vi "dialog.two_button_lua.vi"(5 "LuaVIEW reference":T1) -> (15 "error out":errorcluster)   [LabVIEW 2012]
doc: "Display a two-button dialog with a message. Returns when either button is selected, the dialog window is closed, or the Escape key is pressed. When the left button is selected, the result Boolean returns true. Otherwise false is returned.\n\nThe shown dialog is functionally identical to the standard LabVIEW \"Two Button Dialog\". The standard dialog is not used because, at least up to LabVIEW version 7.1, it has the nasty property that it blocks the user interface thread while open. The UI thread is required not just for display updates but also for VI loading and instantiation. Thus, using the standard \"Two Button Dialog\" might prevent essential background tasks from doing their job.\n\nBeware that the dialog pops up on the machine running Lua, which may not be the same as the machine being operated by the user in case of a client-server setup.\nParameters:\nstr:message. message to display in the dialog box.\nstr:button1, text to display on the left button, e.g. \"OK\".\nstr:button2, text to display on the right button, e.g. \"Cancel\".\nResults:\nbool:confirmed"
uses:
  typedefs/t_LuaVIEW Reference.ctl
  subvis/private/LuaVIEW Pull (string).vi
  subvis/private/LuaVIEW Push (boolean).vi
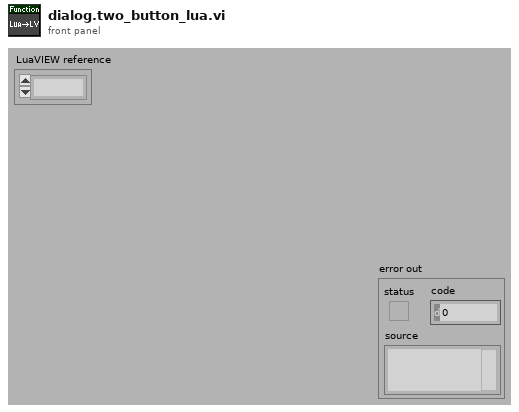
[diagram p1: front panel]
types:
  T1 = typedef "t_LuaVIEW Reference.ctl" = refnum<k1>
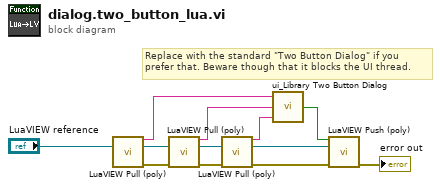
[diagram p0: block diagram]
diagram:
  # "Replace with the standard \"Two Button Dialog\" if you\nprefer that. Beware though that it blocks the UI thread."
  n1 = call-poly "LuaVIEW Pull (poly).vi"("LuaVIEW reference in"="LuaVIEW reference") -> ("string"=w4:string, "LuaVIEW reference out"=w12:T1, "error out"=w3:errorcluster)  [unwired: 12 in]
  n2 = call-poly "LuaVIEW Pull (poly).vi"("LuaVIEW reference in"=w12, "error in (no error)"=w3) -> ("string"=w5:string, "LuaVIEW reference out"=w10:T1, "error out"=w2:errorcluster)  [unwired: 11 in]
  n3 = call-poly "LuaVIEW Pull (poly).vi"("LuaVIEW reference in"=w10, "error in (no error)"=w2) -> ("string"=w6:string, "LuaVIEW reference out"=w8:T1, "error out"=w1:errorcluster)  [unwired: 11 in]
  n4 = call "ui_Library Two Button Dialog.vi"("F button name (\"Cancel\")"=w6, "T button name (\"OK\")"=w5, "message"=w4) -> ("T button?"=w11:bool)
  n5 = call-poly "LuaVIEW Push (poly).vi"("boolean"=w11, "LuaVIEW reference in"=w8, "error in (no error)"=w1) -> ("error out"=→"error out":errorcluster)  [unwired: 11 in, 1 out]
